vi "线性公式.vi"(6 "精度":i32=4, 7 "模型":enum32{"线性", "多项式"}(ring), 8 "method":T1 caption="方法" items=["最小二乘", "最小绝对残差", "Bisquare"], 9 "启用":bool[](array[boolean]), 10 "监测浓度":dbl[](array[numeric]), 11 "标液浓度":dbl[](array[numeric])) -> (1 "XY图":cluster{"X Values":dbl[], "Y Values":dbl[]}[](graph), 2 "r^2":dbl format="%.7g", 3 "拟合方程":string)   [LabVIEW 2016, in "斯坦道总磷总氮.lvlib"]
uses:
  <vilib>/Analysis/6fits.llb/Curve Fitting Criteria.ctl
  <vilib>/Analysis/NI_AALPro.lvlib
  <vilib>/gmath/NI_Gmath.lvlib
panel:
  out "Polynomial Coefficients":dbl[](array[numeric]) caption="多项式系数"
  out "intercept":dbl caption="截距"
  out "slope":dbl caption="斜率"
  out "Best Linear Fit":dbl[](array[numeric]) caption="最佳线性拟合"
  out "二维数组":dbl[][](array[numeric])
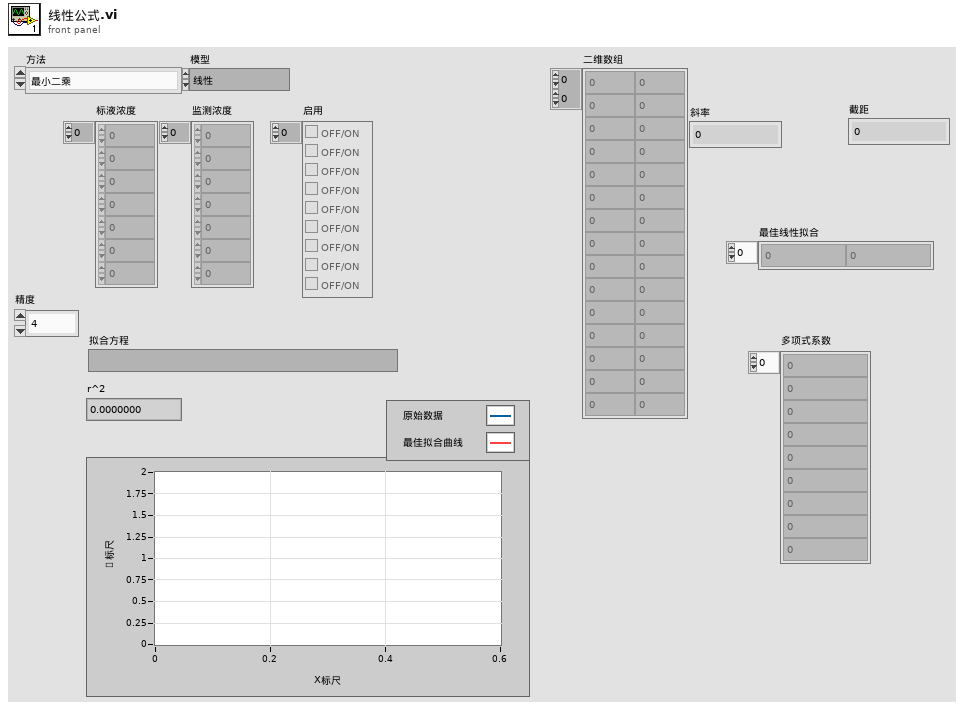
[diagram p1: front panel]
types:
  T1 = typedef "NI_AALPro.lvlib/Curve Fitting Criteria.ctl" = u16
  T2 = enum16{"Linear", "Polynomial", "Exponential", "Power"}
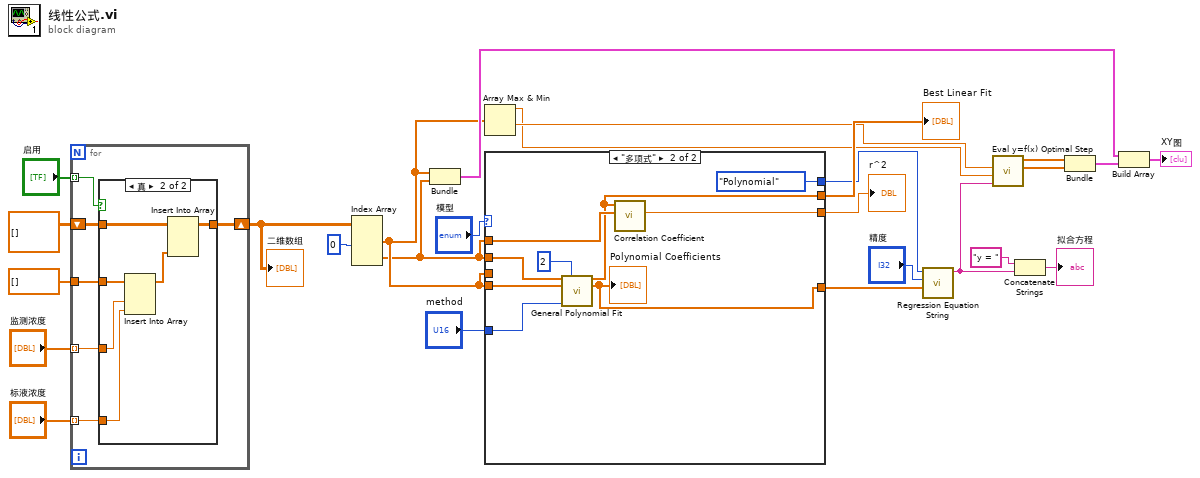
[diagram p0: block diagram]
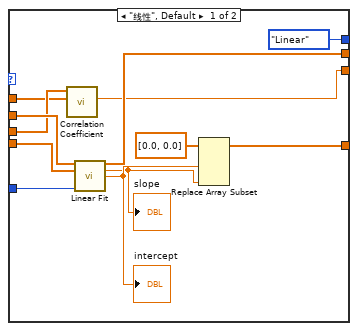
[diagram p2: hidden frame]
diagram:
  n1 = for {
    tunnel: "启用" -> [w27] mode=indexing
    tunnel: "监测浓度" -> [w30] mode=indexing
    tunnel: "标液浓度" -> [w29] mode=indexing
    shift-right: [w28] -> w22
    shift-left: dbl[][] [] ("标液浓度") -> [w32]
    tunnel: dbl[] [] ("监测浓度") -> [w31]
    n2 = case shown="真" w27 {
      tunnel: w32 -> [w33 w39]
      tunnel: w31 -> [_ w38]
      tunnel: w30 -> [_ w37]
      tunnel: w29 -> [_ w36]
      tunnel: [w33 w34] -> w28
      frame False {
      }
      frame True {
        n3 = Insert Into Array(array=w38, new element #1=w37, new element #2=w36) -> (w35:dbl[])  [unwired: 1 in]
        n4 = Insert Into Array(array=w39, new element=w35) -> (w34:dbl[][])  [unwired: 2 in]
      }
    }
  }
  "二维数组" <- w22
  n5 = Index Array(array=w22, index (col) #1=0 ("禁用的索引 (列)")) -> (element #1=w2:dbl[], element #2=w1:dbl[])  [unwired: 3 in]
  n6 = Bundle("标液浓度"=w2, "标液浓度"=w1) -> (w18:cluster{"标液浓度":dbl[], "标液浓度":dbl[]})  [unwired: 1 in]
  n7 = Array Max & Min(array=w2) -> (max value=w6:dbl, min value=w13:dbl)  [unwired: 2 out]
  n8 = case shown="\"多项式\"" "模型" {
    tunnel: [w51 w53] -> w21
    tunnel: "method" -> [w50 w60]
    tunnel: w2 -> [w44 w55]
    tunnel: w1 -> [w43 w56]
    tunnel: [T2."Linear" ("拟合类型") T2."Polynomial" ("拟合类型")] -> w12
    tunnel: [w48 w57] -> w11
    tunnel: [w42 w52] -> w3
    tunnel: w2 -> [w41 _]
    tunnel: w1 -> [w40 w54]
    frame "线性", Default {
      n9 = call <vilib>:"Correlation Coefficient.vi"("Y"=w40, "X"=w41) -> ("r^2"=w42:dbl)  [unwired: 8 in, 1 out]
      n10 = call <vilib>:"Linear Fit.vi"("Y"=w43, "X"=w44, "method"=w50) -> ("Best Linear Fit"=w51:dbl[], "slope"=w45:dbl, "intercept"=w46:dbl)  [unwired: 8 in, 2 out]
      "intercept" <- w46
      "slope" <- w45
      n11 = Replace Array Subset(array=dbl[] [0.0, 0.0] ("数组"), new element #1=w46, new element #2=w45) -> (w48:dbl[])  [unwired: 2 in]
    }
    frame "多项式" {
      n12 = call <vilib>:"General Polynomial Fit.vi"("Y"=w56, "polynomial order"=2, "X"=w55, "method"=w60) -> ("Best Polynomial Fit"=w53:dbl[], "Polynomial Coefficients"=w57:dbl[])  [unwired: 8 in, 2 out]
      "Polynomial Coefficients" <- w57
      n13 = call <vilib>:"Correlation Coefficient.vi"("Y"=w54, "X"=w53) -> ("r^2"=w52:dbl)  [unwired: 8 in, 1 out]
    }
  }
  "Best Linear Fit" <- w21
  "r^2" <- w3
  n14 = call "Regression Equation String.vi"("系数"=w11, "精度"="精度", "拟合类型"=w12) -> ("公式"=w14:string)  [unwired: 8 in]
  n15 = call <vilib>:"Eval y=f(x) Optimal Step.vi"("formula"=w14, "end"=w6, "start"=w13) -> ("Y Values"=w4:dbl[], "X Values"=w16:dbl[])  [unwired: 2 in, 2 out]
  n16 = Concatenate Strings("y = " ("string"), w14) -> (→"拟合方程":string)
  n17 = Bundle("X Values"=w16, "Y Values"=w4) -> (w17:cluster{"X Values":dbl[], "Y Values":dbl[]})  [unwired: 1 in]
  n18 = Build Array(w18, w17) -> (→"XY图":cluster{"X Values":dbl[], "Y Values":dbl[]}[])
